vi "Change_AOM_settings.vi"(8 "VISA Error In":errorcluster) -> (0 "VISA Error Out":errorcluster)   [LabVIEW 2015]
uses:
  <vilib>/Utility/file.llb/Read Delimited Spreadsheet (DBL).vi
  <vilib>/Utility/file.llb/Write Delimited Spreadsheet (DBL).vi
panel:
  in  "Close":bool
  in  "mode":string[](array[string])=["off", "mod", "on", "on", "off", "off", "off", "off"]
  in  "am":i32[](array[numeric])=[0, 400, 715, 340, 0, 0, 0, 0]
  in  "freq":dbl[](array[numeric])=[0.0, 53.105, 75.715, 67.235, 0.0, 0.0, 0.0, 0.0]
  out "chnm":i32[](array[numeric])=[1, 2, 3, 4, 5, 6, 7, 8]
  out "- pin":i32[](array[numeric])=[12, 23, 9, 20, 14, 3, 17, 6]
  out "+ pin":i32[](array[numeric])=[25, 11, 22, 8, 2, 16, 5, 19]
  out "TTL pin":i32[](array[numeric])=[13, 24, 10, 21, 15, 4, 18, 7]
  # "637 nm"
  # "488 nm"
  # "532 nm"
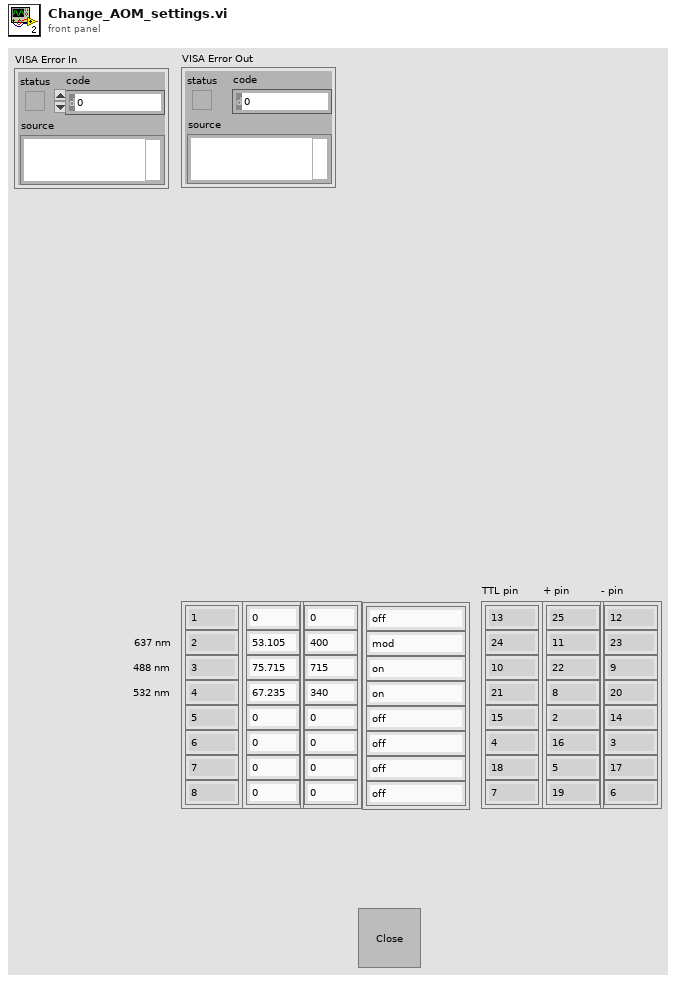
[diagram p1: front panel]
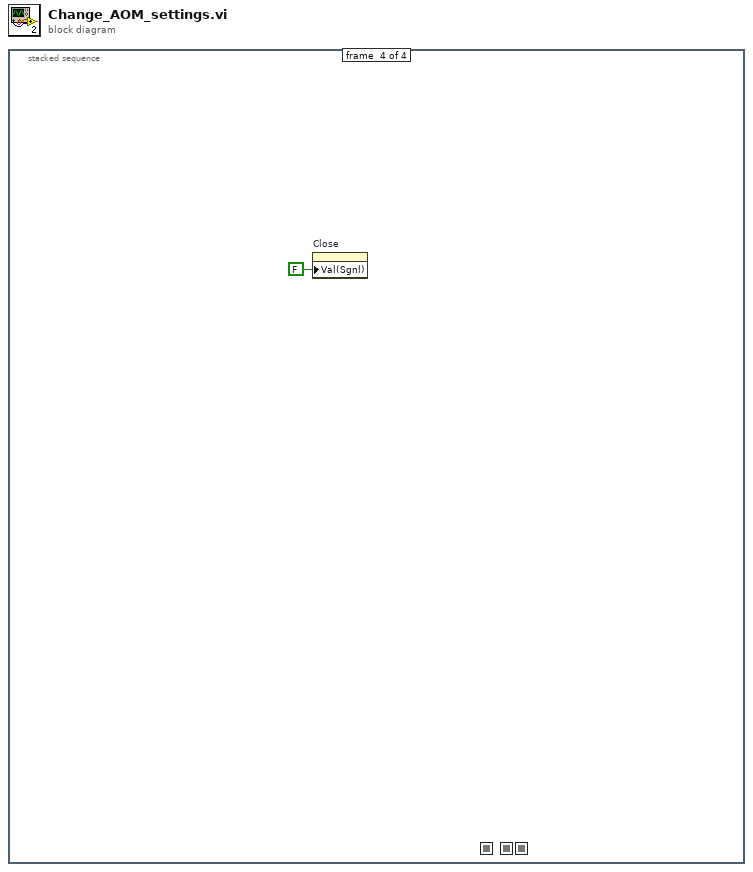
[diagram p0: block diagram]
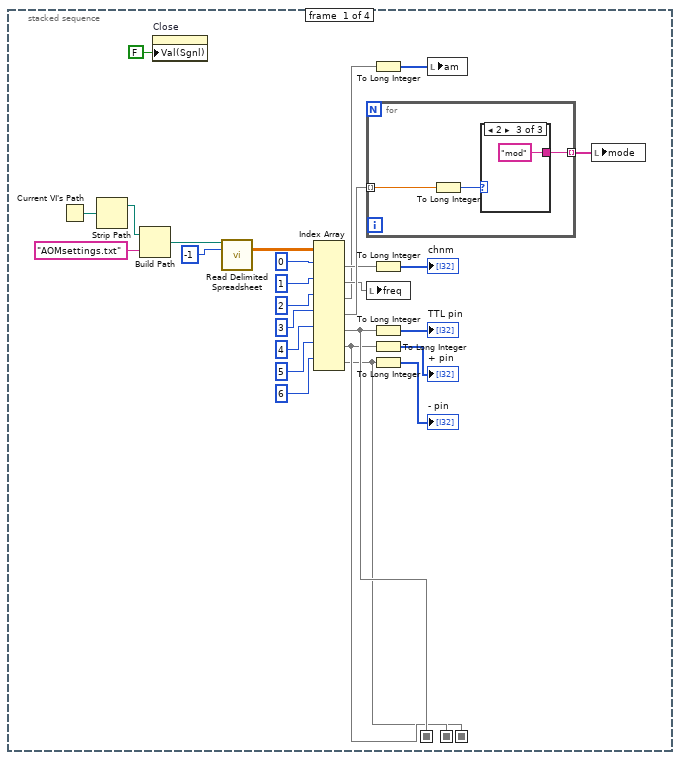
[diagram p2: hidden frame]
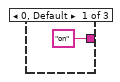
[diagram p3: hidden frame]
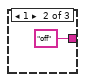
[diagram p4: hidden frame]
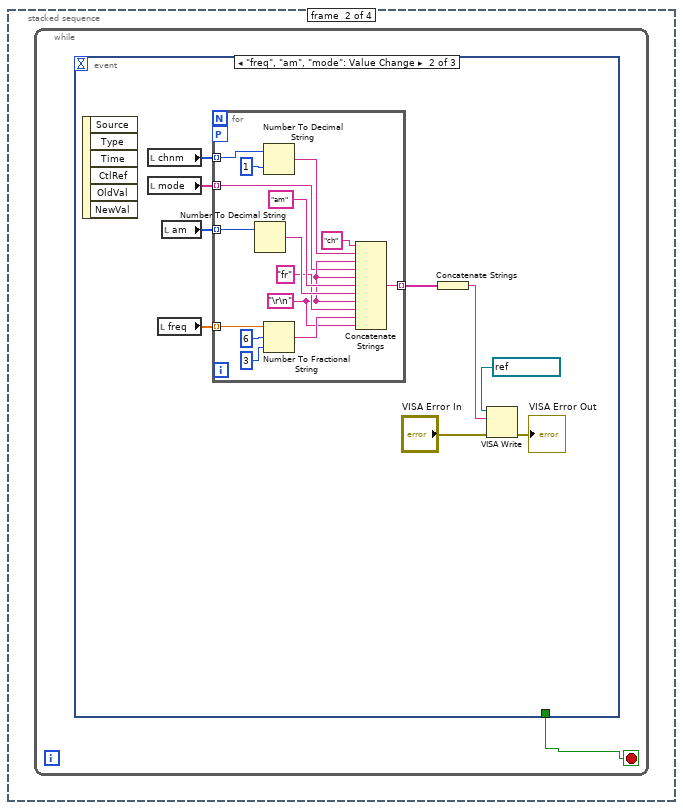
[diagram p5: hidden frame]
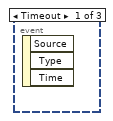
[diagram p6: hidden frame]
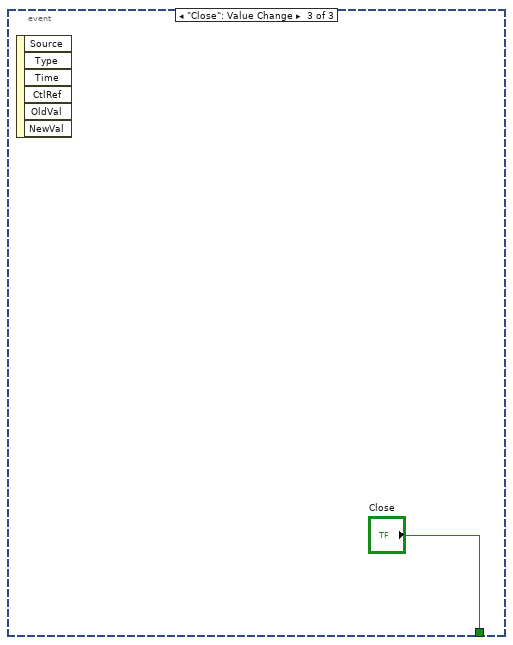
[diagram p7: hidden frame]
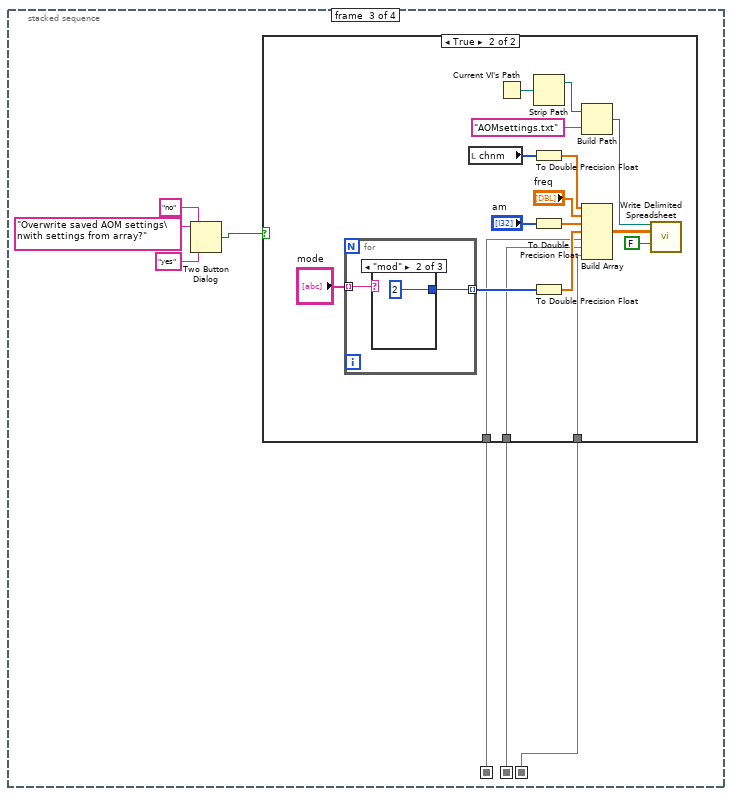
[diagram p8: hidden frame]
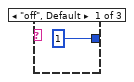
[diagram p10: hidden frame]
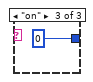
[diagram p11: hidden frame]
diagram:
  n1 = stacked-sequence {
    seq-local: [w7 _ _ _] -> [_ _ w66 _]
    seq-local: [w6 _ _ _] -> [_ _ w65 _]
    seq-local: [w5 _ _ _] -> [_ _ w64 _]
    frame #0 {
      n2 = Current VI's Path() -> (path=w27:path)
      n3 = Strip Path(path=w27) -> (stripped path=w26:path)  [unwired: 1 out]
      n4 = Build Path(base path=w26, name or relative path="AOMsettings.txt") -> (appended path=w24:path)
      n5 = property on="Close" class="Bool (strict)"("Val(Sgnl)"=FALSE ("Value (Signaling)")) -> ()  [unwired: 2 in, 2 out]
      n6 = call-poly <vilib>:"Read Delimited Spreadsheet.vi"("file path (dialog if empty)"=w24, "number of rows (all:-1)"=-1) -> ("all rows"=w22:dbl[][])  [unwired: 8 in, 5 out]
      n7 = Index Array(array=w22, index (row) #1=0 ("index (row)"), index (row) #2=1 ("index (row)"), index (row) #3=2 ("index (row)"), index (row) #4=3 ("index (row)"), index (row) #5=4 ("index (row)"), index (row) #6=5 ("index (row)"), index (row) #7=6 ("index (row)")) -> (element #1=w15:dbl[], element #2=w14:dbl[], element #3=w13:dbl[], element #4=w17:dbl[], element #5=w7:dbl[], element #6=w6:dbl[], element #7=w5:dbl[])  [unwired: 7 in]
      n8 = for {
        tunnel: w17 -> [w30] mode=indexing
        tunnel: [w29] -> w16 mode=indexing
        n9 = To Long Integer(number=w30) -> (32bit integer=w28:i32)
        n10 = case shown="2" w28 {
          tunnel: ["on" "off" "mod"] -> w29
          frame 0, Default {
          }
          frame 1 {
          }
          frame 2 {
          }
        }
      }
      n11 = local write "freq"(w14) -> ()
      n12 = To Long Integer(number=w13) -> (32bit integer=w11:i32[])
      n13 = To Long Integer(number=w15) -> (32bit integer=→"chnm":i32[])
      n14 = To Long Integer(number=w7) -> (32bit integer=→"TTL pin":i32[])
      n15 = To Long Integer(number=w6) -> (32bit integer=→"+ pin":i32[])
      n16 = To Long Integer(number=w5) -> (32bit integer=→"- pin":i32[])
      n17 = local write "am"(w11) -> ()
      n18 = local write "mode"(w16) -> ()
    }
    frame #1 {
      n19 = while {
        stop <- w34 stop-if-true
        n20 = event shown="[1] \"freq\", \"am\", \"mode\": Value Change" {
          selector: _ -> [_ _ _]
          dyn-events: _ -> [_ _ _]
          timeout: _ -> [_ _ _]
          tunnel: [_ _ "Close"] -> w34
          event Timeout {
            n21 = event-data() -> ()  [unwired: 1 in, 3 out]
          }
          event "freq", "am", "mode": Value Change {
            n22 = event-data() -> ()  [unwired: 1 in, 6 out]
            n23 = local read "chnm"() -> (w40:i32[])
            n24 = local read "mode"() -> (w43:string[])
            n25 = local read "freq"() -> (w41:dbl[])
            n26 = local read "am"() -> (w42:i32[])
            n27 = for {
              workers-P: _ -> [_]
              tunnel: w40 -> [w50] mode=indexing
              tunnel: w41 -> [w48] mode=indexing
              tunnel: w42 -> [w49] mode=indexing
              tunnel: [w47] -> w39 mode=indexing
              tunnel: w43 -> [w44] mode=indexing
              w51 = "\r\n"
              n28 = Number To Decimal String(number=w49) -> (decimal integer string=w54:string)  [unwired: 1 in]
              n29 = Number To Decimal String(number=w50, width (-)=i16 1) -> (decimal integer string=w46:string)
              n30 = Number To Fractional String(number=w48, width (-)=i16 6, precision (6)=i16 3) -> (F-format string=w52:string)  [unwired: 1 in]
              n31 = Concatenate Strings("ch", w46, w51, w44, w51, "am", w54, w51, "fr", w52, w51) -> (w47:string)
            }
            n32 = Concatenate Strings(w39) -> (w37:string)
            n33 = VISA Write(VISA resource name=refnum<visa-resource-name> "COM13" ("COM channel"), write buffer=w37, error in (no error)="VISA Error In") -> (error out=→"VISA Error Out":errorcluster)  [unwired: 2 out]
          }
          event "Close": Value Change {
            n34 = event-data() -> ()  [unwired: 1 in, 6 out]
          }
        }
      }
    }
    frame #2 {
      n35 = Two Button Dialog(message="Overwrite saved AOM settings\nwith settings from array?", 1:"no" ("F button name (\"Cancel\")"), 2:"yes" ("T button name (\"OK\")")) -> (T button?=w63:bool)
      n36 = case shown="True" w63 {
        tunnel: w66 -> [_ w69]
        tunnel: w65 -> [_ w68]
        tunnel: w64 -> [_ w67]
        frame False {
        }
        frame True {
          n37 = for {
            tunnel: "mode" -> [w85] mode=indexing
            tunnel: [w84] -> w80 mode=indexing
            n38 = case shown="\"mod\"" w85 {
              tunnel: [1 2 0] -> w84
              frame "off", Default {
              }
              frame "mod" {
              }
              frame "on" {
              }
            }
          }
          n39 = local read "chnm"() -> (w70:i32[])
          n40 = Current VI's Path() -> (path=w77:path)
          n41 = Strip Path(path=w77) -> (stripped path=w76:path)  [unwired: 1 out]
          n42 = To Double Precision Float(number=w70) -> (double precision float=w79:dbl[])
          n43 = To Double Precision Float(number="am") -> (double precision float=w71:dbl[])
          n44 = To Double Precision Float(number=w80) -> (double precision float=w78:dbl[])
          n45 = Build Path(base path=w76, name or relative path="AOMsettings.txt") -> (appended path=w74:path)
          n46 = Build Array(w79, "freq", w71, w78, w69, w68, w67) -> (w73:dbl[][])
          n47 = call-poly <vilib>:"Write Delimited Spreadsheet.vi"("file path (dialog if empty)"=w74, "2D data"=w73, "append to file? (F)"=FALSE) -> ()  [unwired: 11 in, 2 out]
        }
      }
    }
    frame #3 {
      n48 = property on="Close" class="Bool (strict)"("Val(Sgnl)"=FALSE ("Value (Signaling)")) -> ()  [unwired: 2 in, 2 out]
    }
  }
